vi "DB Delete.vi"(6 "Where":string, 7 "table Name":string, 8 "error in (no error)":errorcluster, 11 "Db Reference":refnum<k24>) -> (0 "error out":errorcluster, 3 "Db Reference":refnum<k24>)   [LabVIEW 2020]
uses:
  D:/Labview/Auto Run Screen/Source Code/Database/Support/dbquery.dll
  Support/dbquery.dll
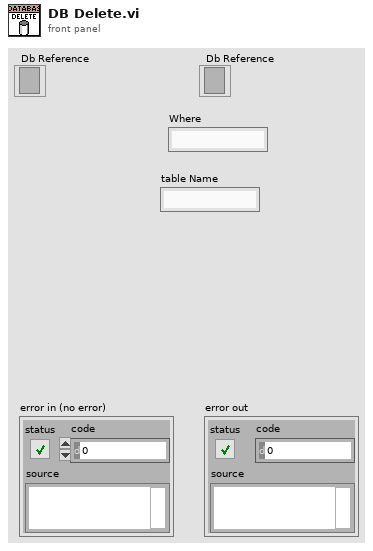
[diagram p1: front panel]
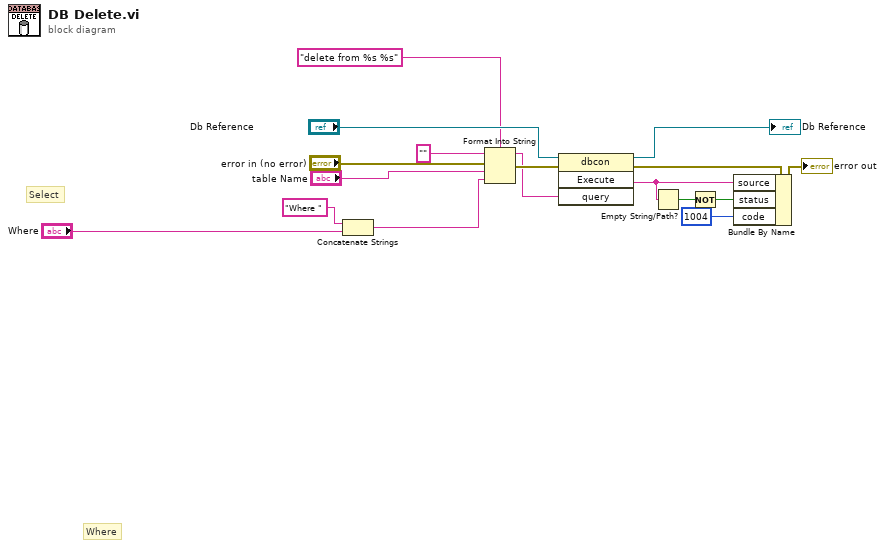
[diagram p0: block diagram]
diagram:
  # "Where"
  # "Select"
  n1 = Concatenate Strings("Where " ("string"), "Where") -> (w6:string)
  n2 = Format Into String(format string="delete from %s %s", initial string="", error in="error in (no error)", "table Name", w6) -> (resulting string=w10:string, error out=w11:errorcluster)
  n3 = invoke class="dbcon" method="Execute"(reference="Db Reference", error in=w11, "query"=w10) -> (reference out=→"Db Reference":refnum<k24>, error out=w7:errorcluster, "Execute"=w4:string)  [unwired: 1 in, 1 out]
  n4 = Empty String/Path?(string/path=w4) -> (empty?=w3:bool)
  n5 = Not(x=w3) -> (.not. x?=w2:bool)
  n6 = Bundle By Name(cluster=w7, "source"=w4, "status"=w2, "code"=1004) -> (→"error out":errorcluster)
